vi "Get Active Memory.vi"(0 "VISA resource name":refnum<visa-resource-name>, 11 "error in (no error)":errorcluster) -> (4 "VISA resource name out":refnum<visa-resource-name>, 6 "Memory":i32, 15 "error out":errorcluster)   [LabVIEW 2014, in "eec 6700.lvlib"]
doc: "Gets the Active Memory set to the Power source instrument."
uses:
  <instrlib>/eec 6700/eec 6700.lvlib
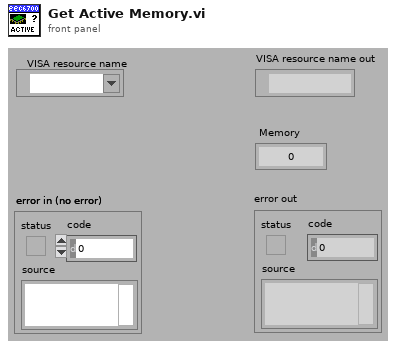
[diagram p1: front panel]
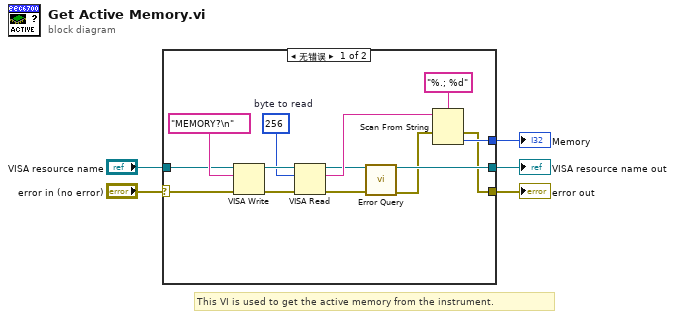
[diagram p0: block diagram]
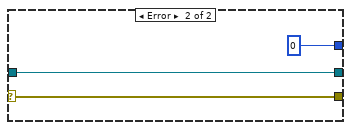
[diagram p2: hidden frame]
diagram:
  # "This VI is used to get the active memory from the instrument."
  n1 = case shown="无错误" "error in (no error)" {
    selector: "error in (no error)" -> [w18 w22]
    tunnel: [w7 w22] -> w4
    tunnel: [w9 w21] -> w2
    tunnel: "VISA resource name" -> [w17 w21]
    tunnel: [w14 0] -> w1
    frame No Error {
      w11 = u32 256  # byte to read
      n2 = VISA Write(VISA resource name=w17, write buffer="MEMORY?\n", error in (no error)=w18) -> (VISA resource name out=w13:refnum<visa-resource-name>, error out=w12:errorcluster)  [unwired: 1 out]
      n3 = VISA Read(VISA resource name=w13, byte count=w11, error in (no error)=w12) -> (VISA resource name out=w10:refnum<visa-resource-name>, read buffer=w16:string, error out=w8:errorcluster)  [unwired: 1 out]
      n4 = call <instrlib>:"Error Query.vi"("VISA resource name"=w10, "error in (no error)"=w8) -> ("VISA resource name out"=w9:refnum<visa-resource-name>, "error out"=w6:errorcluster)  [unwired: 10 in, 2 out]
      n5 = Scan From String(format string="%.; %d", input string=w16, error in=w6) -> (error out=w7:errorcluster, output 1=w14:i32)  [unwired: 2 in, 2 out]
    }
    frame Error {
    }
  }
  "error out" <- w4
  "VISA resource name out" <- w2
  "Memory" <- w1
